vi "Generate Query Command.vi"(8 "Error In":errorcluster, 10 "Coordenates":T1 {"Longitude" format="%#_13g"; "Latitude" format="%#_13g"}, 11 "Open Weather Session In":refnum<class "Open Weather Session.lvclass">) -> (0 "Error Out":errorcluster, 1 "Query Command":string, 3 "Open Weather Session Out":refnum<class "Open Weather Session.lvclass">)   [LabVIEW 2019, in "Open Weather Session.lvclass"]
uses:
  Open Weather Session.lvclass
  Public/Controls/Coordenates.ctl
  Accessors/API Key/Get API Key.vi
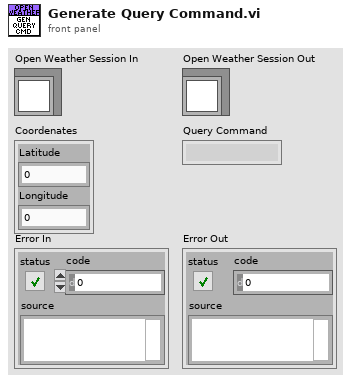
[diagram p1: front panel]
types:
  T1 = typedef "Open Weather Session.lvclass/Coordenates.ctl" = cluster{"Latitude":dbl, "Longitude":dbl}
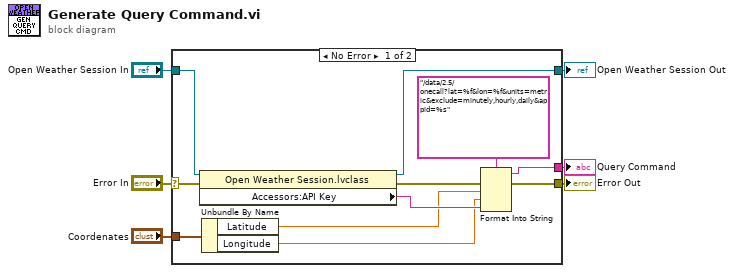
[diagram p0: block diagram]
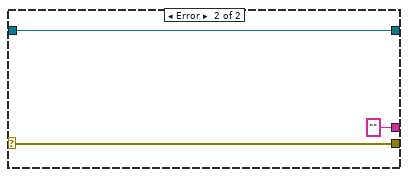
[diagram p2: hidden frame]
diagram:
  n1 = case shown="No Error" "Error In" {
    selector: "Error In" -> [w11 w19]
    tunnel: [w17 w20] -> w6
    tunnel: [w15 w19] -> w5
    tunnel: [w13 ""] -> w4
    tunnel: "Open Weather Session In" -> [w10 w20]
    tunnel: "Coordenates" -> [w9 _]
    frame No Error {
      n2 = property class="Open Weather Session.lvclass"(reference=w10, error in=w11) -> (reference out=w17:refnum<class "Open Weather Session.lvclass">, error out=w14:errorcluster, "Accessors:API Key"=w16:string)
      n3 = Unbundle By Name(w9) -> ("Latitude"=w8:dbl, "Longitude"=w7:dbl)
      n4 = Format Into String(format string="/data/2.5/onecall?lat=%f&lon=%f&units=metric&exclude=minutely,hourly,daily&appid=%s", error in=w14, w8, w7, w16) -> (resulting string=w13:string, error out=w15:errorcluster)  [unwired: 1 in]
    }
    frame Error {
    }
  }
  "Open Weather Session Out" <- w6
  "Error Out" <- w5
  "Query Command" <- w4
